vi "get_errors.vi"(0 "HGF_FGV_Visitor":refnum<class "HGF_FGV_Visitor.lvclass">, 5 "error in (no error)":errorcluster) -> (14 "dup HGF_FGV_Visitor":refnum<class "HGF_FGV_Visitor.lvclass">, 16 "Errors":errorcluster[](array[cluster]), 17 "error":bool, 19 "error out":errorcluster)   [LabVIEW 2012, in "HGF_FGV.lvlib" / "HGF_FGV_Visitor.lvclass"]
uses:
  HGF_FGV_Visitor.lvclass
  HGF_FGV_Visitor.lvclass/HGF_FGV_Visitor.ctl
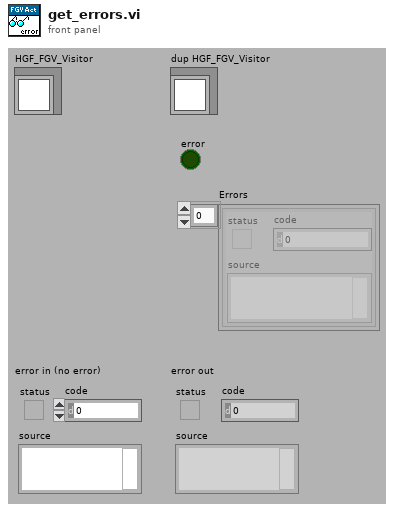
[diagram p1: front panel]
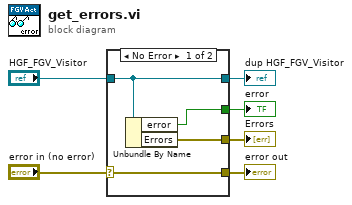
[diagram p0: block diagram]
diagram:
  n1 = case shown="No Error" "error in (no error)" {
    selector: "error in (no error)" -> [w10 w11]
    tunnel: [w10 w11] -> w5
    tunnel: [w9 w12] -> w3
    tunnel: "HGF_FGV_Visitor" -> [w9 w12]
    tunnel: [w8 _] -> w2
    tunnel: [w7 _] -> w1
    frame No Error {
      n2 = Unbundle By Name(w9) -> ("error"=w7:bool, "Errors"=w8:errorcluster[])
    }
    frame Error {
    }
  }
  "error out" <- w5
  "dup HGF_FGV_Visitor" <- w3
  "Errors" <- w2
  "error" <- w1
